vi "DLPConfigInitialization_XML_Read.vi"(8 "error in (no error)":errorcluster, 11 "Recipe XML File Path":path) -> (0 "error out":errorcluster, 2 "DLP":T1)   [LabVIEW 2022 SP3]
uses:
  Controls/DLPConfig_Initialization.ctl
  Classes/DLP2/DataTypes/DLP2_PrinterCompensationProperties.ctl
  Classes/DLP2/DataTypes/DLP2_PrinterHeadProperties.ctl
  Controls/DLPConfig)Init_HeadPropertyAttr--Cluster.ctl
  Classes/DLP2/DataTypes/DLP2_PrinterMaterialProperties.ctl
  Classes/TopLevel/Typedefs/InkIdleNodeConfigXML--Cluster.ctl
  Classes/TopLevel/Typedefs/InkProcessNodeConfigXML--Cluster.ctl
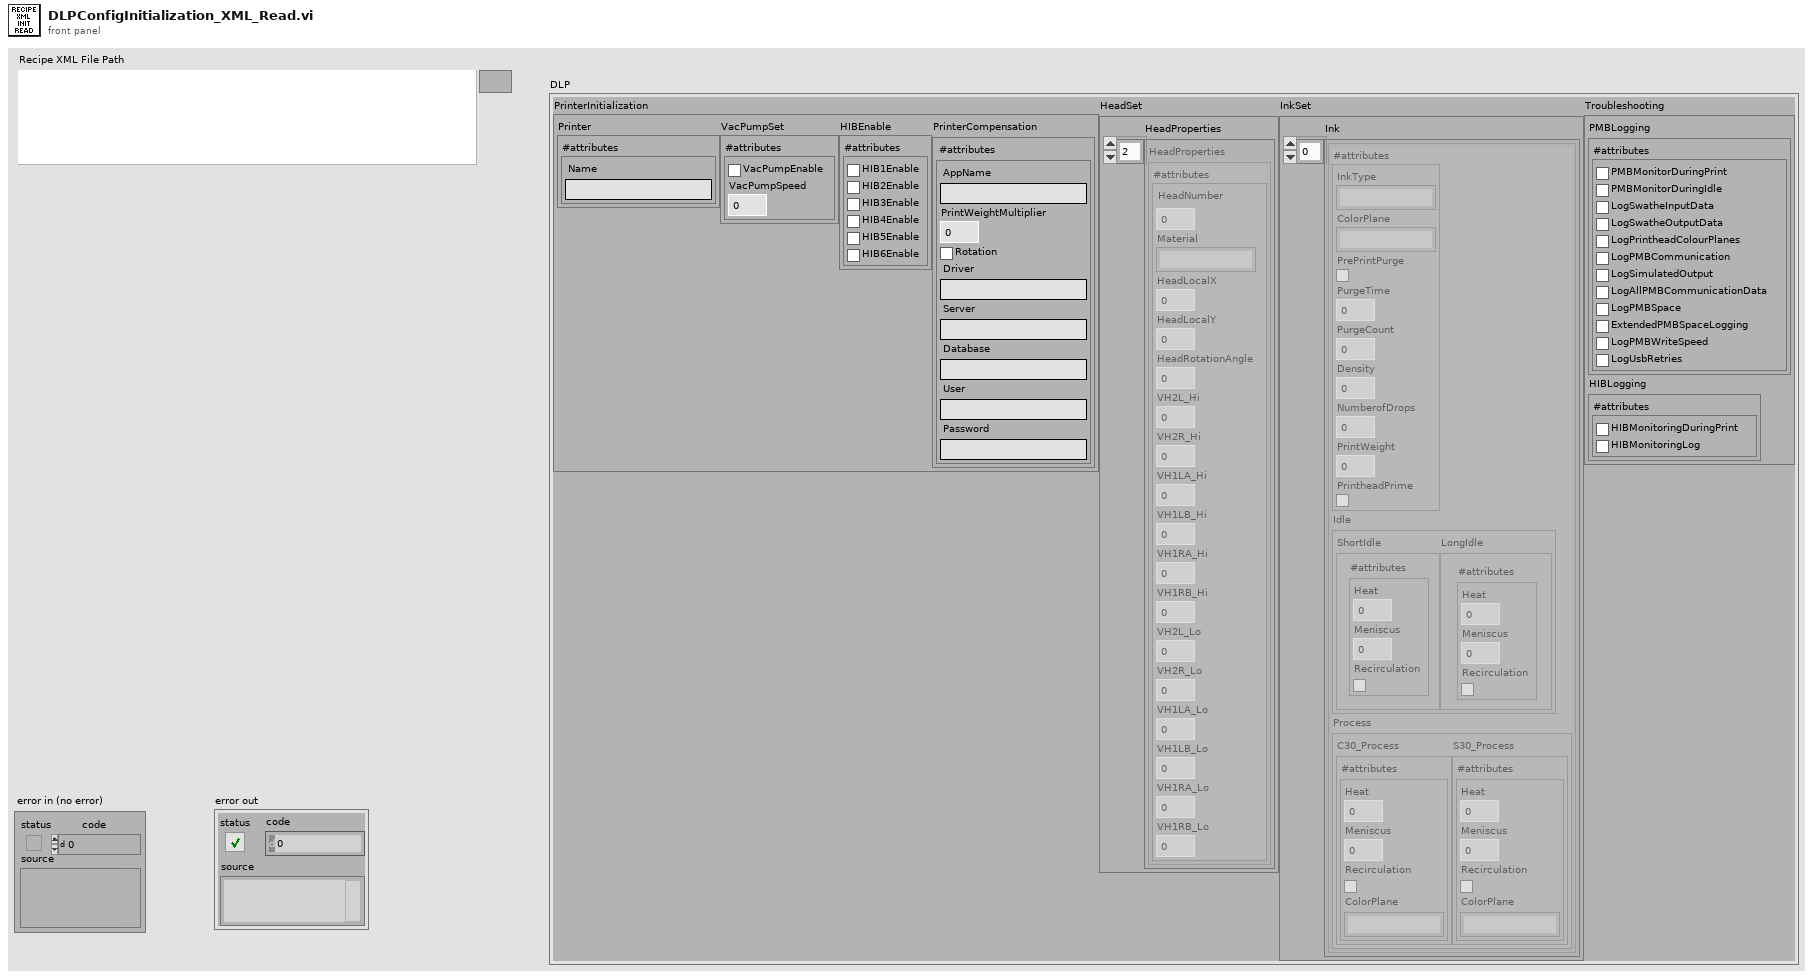
[diagram p1: front panel]
types:
  T1 = typedef "DLPConfig_Initialization.ctl" = cluster{"PrinterInitialization":cluster{"Printer":cluster{"#attributes":cluster{"Name":string}}, "VacPumpSet":cluster{"#attributes":cluster{"VacPumpEnable":bool, "VacPumpSpeed":dbl}}, "HIBEnable":cluster{"#attributes":cluster{"HIB1Enable":bool, "HIB2Enable":bool, "HIB3Enable":bool, "HIB4Enable":bool, "HIB5Enable":bool, "HIB6Enable":bool}}, "PrinterCompensation":T2}, "HeadSet":cluster{"HeadProperties":T3[]}, "InkSet":cluster{"Ink":T5[]}, "Troubleshooting":cluster{"PMBLogging":cluster{"#attributes":cluster{"PMBMonitorDuringPrint":bool, "PMBMonitorDuringIdle":bool, "LogSwatheInputData":bool, "LogSwatheOutputData":bool, "LogPrintheadColourPlanes":bool, "LogPMBCommunication":bool, "LogSimulatedOutput":bool, "LogAllPMBCommunicationData":bool, "LogPMBSpace":bool, "ExtendedPMBSpaceLogging":bool, "LogPMBWriteSpeed":bool, "LogUsbRetries":bool}}, "HIBLogging":cluster{"#attributes":cluster{"HIBMonitoringDuringPrint":bool, "HIBMonitoringLog":bool}}}}
  T2 = typedef "DLP2_PrinterCompensationProperties.ctl" = cluster{"#attributes":cluster{"AppName":string, "PrintWeightMultiplier":dbl, "Rotation":bool, "Driver":string, "Server":string, "Database":string, "User":string, "Password":string}}
  T3 = typedef "DLP2_PrinterHeadProperties.ctl" = cluster{"#attributes":T4}
  T4 = typedef "DLPConfig)Init_HeadPropertyAttr--Cluster.ctl" = cluster{"HeadNumber":u8, "Material":string, "HeadLocalX":dbl, "HeadLocalY":dbl, "HeadRotationAngle":dbl, "VH2L_Hi":dbl, "VH2R_Hi":dbl, "VH1LA_Hi":dbl, "VH1LB_Hi":dbl, "VH1RA_Hi":dbl, "VH1RB_Hi":dbl, "VH2L_Lo":dbl, "VH2R_Lo":dbl, "VH1LA_Lo":dbl, "VH1LB_Lo":dbl, "VH1RA_Lo":dbl, "VH1RB_Lo":dbl}
  T5 = typedef "DLP2_PrinterMaterialProperties.ctl" = cluster{"#attributes":cluster{"InkType":string, "ColorPlane":string, "PrePrintPurge":bool, "PurgeTime":dbl, "PurgeCount":i32, "Density":dbl, "NumberofDrops":i32, "PrintWeight":dbl, "PrintheadPrime":bool}, "Idle":T6, "Process":T7}
  T6 = typedef "InkIdleNodeConfigXML--Cluster.ctl" = cluster{"ShortIdle":cluster{"#attributes":cluster{"Heat":dbl, "Meniscus":dbl, "Recirculation":bool}}, "LongIdle":cluster{"#attributes":cluster{"Heat":dbl, "Meniscus":dbl, "Recirculation":bool}}}
  T7 = typedef "InkProcessNodeConfigXML--Cluster.ctl" = cluster{"C30_Process":cluster{"#attributes":cluster{"Heat":dbl, "Meniscus":dbl, "Recirculation":bool, "ColorPlane":string}}, "S30_Process":cluster{"#attributes":cluster{"Heat":dbl, "Meniscus":dbl, "Recirculation":bool, "ColorPlane":string}}}
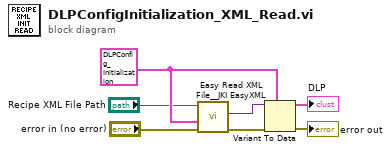
[diagram p0: block diagram]
diagram:
  w2 = T1 {"PrinterInitialization"={"Printer"={"#attributes"={"Name"=""}}, "VacPumpSet"={"#attributes"={"VacPumpEnable"=FALSE, "VacPumpSpeed"=0.0}}, "HIBEnable"={"#attributes"={"HIB1Enable"=FALSE, "HIB2Enable"=FALSE, "HIB3Enable"=FALSE, "HIB4Enable"=FALSE, "HIB5Enable"=FALSE, "HIB6Enable"=FALSE}}, "PrinterCompensation"={"#attributes"={"AppName"="", "PrintWeightMultiplier"=0.0, "Rotation"=FALSE, "Driver"="", "Server"="", "Database"="", "User"="", "Password"=""}}}, "HeadSet"={"HeadProperties"=[]}, "InkSet"={"Ink"=[]}, "Troubleshooting"={"PMBLogging"={"#attributes"={"PMBMonitorDuringPrint"=FALSE, "PMBMonitorDuringIdle"=FALSE, "LogSwatheInputData"=FALSE, "LogSwatheOutputData"=FALSE, "LogPrintheadColourPlanes"=FALSE, "LogPMBCommunication"=FALSE, "LogSimulatedOutput"=FALSE, "LogAllPMBCommunicationData"=FALSE, "LogPMBSpace"=FALSE, "ExtendedPMBSpaceLogging"=FALSE, "LogPMBWriteSpeed"=FALSE, "LogUsbRetries"=FALSE}}, "HIBLogging"={"#attributes"={"HIBMonitoringDuringPrint"=FALSE, "HIBMonitoringLog"=FALSE}}}} ("DLP")
  n1 = call <vilib>:"Easy Read XML File__JKI EasyXML.vi"("error in (no error)"="error in (no error)", "LabVIEW Data (Type)"=w2, "XML File Path"="Recipe XML File Path") -> ("error out"=w5:errorcluster, "LabVIEW Data"=w6:variant)  [unwired: 6 in, 1 out]
  n2 = Variant To Data(error in=w5, type=w2, Variant=w6) -> (data=→"DLP":T1, error out=→"error out":errorcluster)
